vi "5.vi"() -> ()   [LabVIEW 2023]
uses:
  <vilib>/Analysis/NI_AALPro.lvlib
panel:
  in  "?":bool
  out "b calculat":dbl
  out "a calculat":dbl
  in  "Eroare[%]":dbl(slide) scale=0.0..20.0
  in  "b":dbl(slide) scale=-10.0..10.0
  in  "a":dbl(slide) scale=-10.0..10.0
  out "XY Graph":cluster{i32[], dbl[]}[](graph)
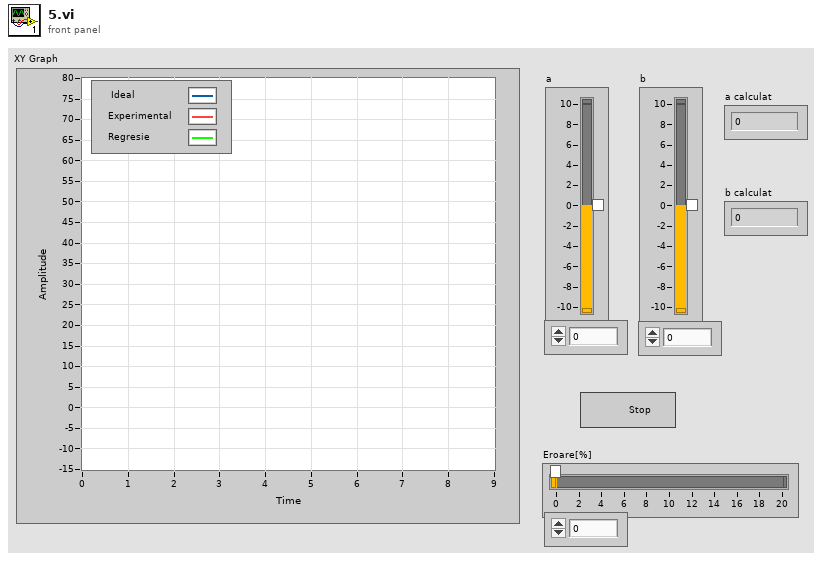
[diagram p1: front panel]
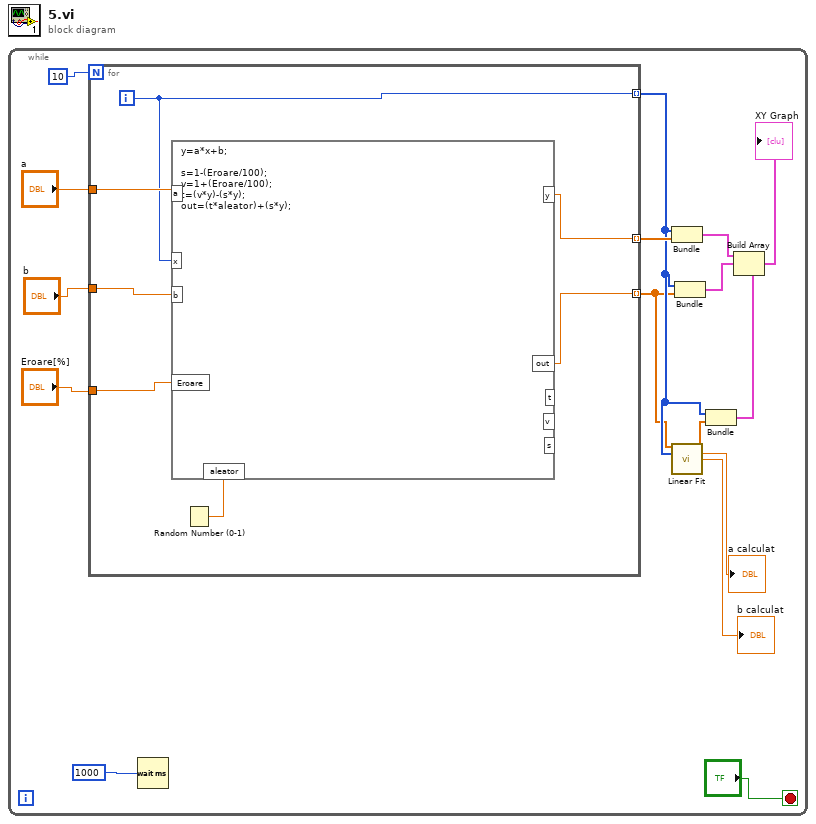
[diagram p0: block diagram]
diagram:
  n1 = while {
    stop <- "?" stop-if-true
    n2 = for {
      N: 10 -> [_]
      tunnel: "a" -> [w23]
      tunnel: "b" -> [w22]
      tunnel: "Eroare[%]" -> [w21]
      tunnel: [w18] -> w3 mode=indexing
      tunnel: [w20] -> w4 mode=indexing
      tunnel: [w19] -> w2 mode=indexing
      i -> [w18]
      n3 = Random Number (0-1)() -> (number: 0 to 1=w17:dbl)
      n4 = formula code="y=a*x+b;\n\ns=1-(Eroare/100);\nv=1+(Eroare/100);\nt=(v*y)-(s*y);\nout=(t*aleator)+(s*y);"("a"=w23, "b"=w22, "Eroare"=w21, "x"=w18, "aleator"=w17) -> ("y"=w20:dbl, "out"=w19:dbl)  [unwired: 3 out]
    }
    n5 = Wait (ms)(milliseconds to wait=1000) -> ()  [unwired: 1 out]
    n6 = Bundle(w3, w4) -> (w11:cluster{i32[], dbl[]})  [unwired: 1 in]
    n7 = call <vilib>:"Linear Fit.vi"("Y"=w2, "X"=w3) -> ("Best Linear Fit"=w1:dbl[], "slope"=→"a calculat":dbl, "intercept"=→"b calculat":dbl)  [unwired: 9 in, 2 out]
    n8 = Bundle(w3, w2) -> (w10:cluster{i32[], dbl[]})  [unwired: 1 in]
    n9 = Bundle(w3, "Best Linear Fit"=w1) -> (w9:cluster{i32[], "Best Linear Fit":dbl[]})  [unwired: 1 in]
    n10 = Build Array(w11, w10, w9) -> (→"XY Graph":cluster{i32[], "Best Linear Fit":dbl[]}[])
  }
